vi "save_s1p_file.vi"(8 "button_save_s1p":bool, 10 "data_array_in":dbl[][](array[numeric]), 11 "freq_array_in":dbl[](array[numeric])) -> ()   [LabVIEW 2025]
panel:
  out "Save Buffer":string
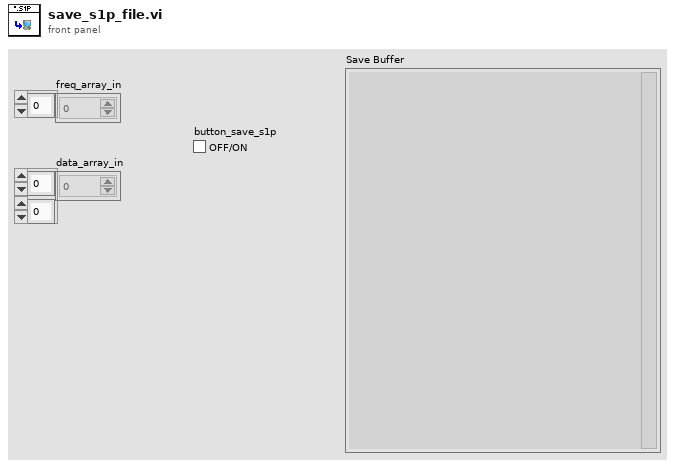
[diagram p1: front panel]
types:
  T1 = enum16{"open", "replace", "create", "open or create", "replace or create", "replace or create with confirmation"}
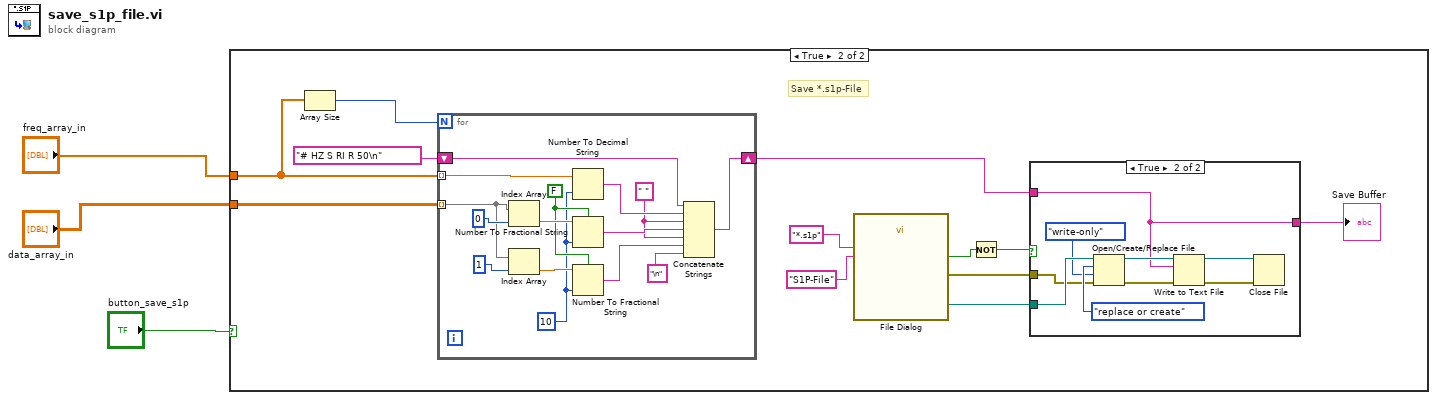
[diagram p0: block diagram]
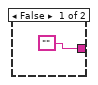
[diagram p3: hidden frame]
diagram:
  n1 = case shown="True" "button_save_s1p" {
    tunnel: "freq_array_in" -> [_ w5]
    tunnel: "data_array_in" -> [_ w14]
    frame False {
    }
    frame True {
      # "Save *.s1p-File"
      n2 = Array Size(array=w5) -> (size(s)=w4:i32)
      n3 = for {
        N: w4 -> [_]
        shift-right: [w32] -> w9
        shift-left: "# HZ S RI R 50\n" -> [w31]
        tunnel: w5 -> [w30] mode=indexing
        tunnel: w14 -> [w29] mode=indexing
        w26 = i16 10 ("precision (6)")
        w33 = FALSE ("use system decimal point (T)")
        w28 = " " ("string")
        n4 = Index Array(array=w29, index=0 ("index (col)")) -> (element=w37:dbl)
        n5 = Index Array(array=w29, index=1 ("index (col)")) -> (element=w35:dbl)
        n6 = Number To Decimal String(number=w30, width (-)=w26) -> (decimal integer string=w38:string)
        n7 = Number To Fractional String(use system decimal point (T)=w33, number=w37, precision (6)=w26) -> (F-format string=w36:string)  [unwired: 1 in]
        n8 = Number To Fractional String(use system decimal point (T)=w33, number=w35, precision (6)=w26) -> (F-format string=w34:string)  [unwired: 1 in]
        n9 = Concatenate Strings(w31, w38, w28, w36, w28, w34, "\n" ("string")) -> (w32:string)
      }
      n10 = call "File Dialog"("pattern (all files)"="*.s1p" ("pattern label"), "pattern label"="S1P-File") -> ("selected path"=w11:path, "cancelled"=w7:bool, "error out"=w10:errorcluster)  [unwired: 10 in, 1 out]
      n11 = Not(x=w7) -> (.not. x?=w8:bool)
      n12 = case shown="True" w8 {
        tunnel: w11 -> [_ w24]
        tunnel: w10 -> [_ w23]
        tunnel: w9 -> [_ w17]
        tunnel: ["" w17] -> w6
        frame False {
        }
        frame True {
          n13 = Open/Create/Replace File(file path (use dialog)=w24, error in=w23, operation (0:open)=T1."replace or create", access (0:read/write)=enum16{"read/write", "read-only", "write-only"}."write-only") -> (refnum out=w22:refnum<file>, error out=w21:errorcluster)  [unwired: 2 in, 1 out]
          n14 = Write to Text File(file (use dialog)=w22, text=w17, error in=w21) -> (refnum out=w19:refnum<file>, error out=w20:errorcluster)  [unwired: 1 in, 1 out]
          n15 = Close File(refnum=w19, error in=w20) -> ()  [unwired: 2 out]
        }
      }
      "Save Buffer" <- w6
    }
  }
